vi "ex_GetHeader.vi"(0 "file path":path, 1 "file refs in":T1={"file ref"=refnum, "file size (bytes:0)"=0, "read pointer (bytes:0)"=0, "chunk size (bytes:65000)"=65000}, 2 "file dialog?":bool, 7 "chunk in":string, 9 "first_time?":bool, 11 "error in (no error)":errorcluster) -> (3 "Decimal Separator":string, 4 "hdr special blks":string[](array[string]), 6 "optional info":T3, 8 "file_params":T2 {"time preference" items=["Absolute", "Relative"]; "x_columns" items=["None", "One", "Multiple"]}, 10 "delimiter":string, 12 "chunk remainder":string, 13 "file refs out":T1, 14 "origin timestamp":timestamp format="%<%X\n%x>T", 15 "error out":errorcluster)   [LabVIEW 2020]
uses:
  <vilib>/express/express shared/ExFile.llb/ex_FileReference.ctl
  <vilib>/express/express input/ExFileReadBlock.llb/ex_ReadFileParams.ctl
  <vilib>/express/express shared/ExFile.llb/ex_FileGlobals.vi
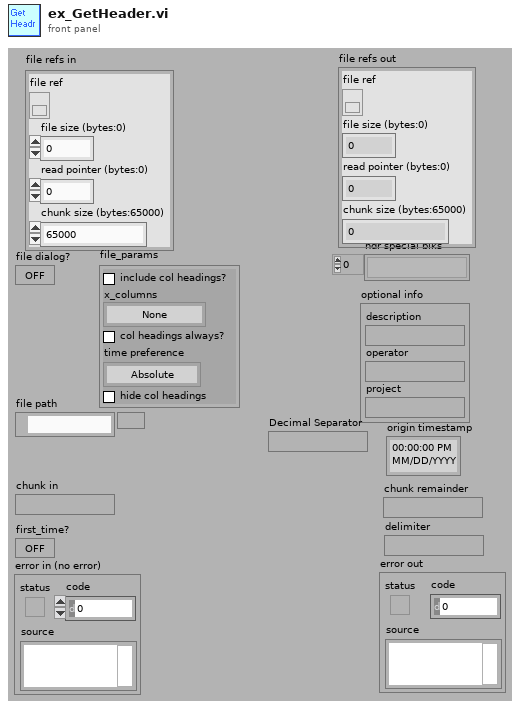
[diagram p1: front panel]
types:
  T1 = typedef "ex_FileReference.ctl" = cluster{"file ref":refnum<file>, "file size (bytes:0)":i32, "read pointer (bytes:0)":i32, "chunk size (bytes:65000)":i32}
  T2 = typedef "ex_ReadFileParams.ctl" = cluster{"include col headings?":bool, "x_columns":u16, "col headings always?":bool, "time preference":u16, "hide col headings":bool}
  T3 = cluster{"description":string, "operator":string, "project":string}
  T4 = enum32{"existing file", "new file", "new or existing file", "existing dir", "new dir", "new or existing dir", "existing file (use LLBs)", "new file (use LLBs)", "new or existing file (use LLBs)", "new or existing file or directory (use LLBs)"}
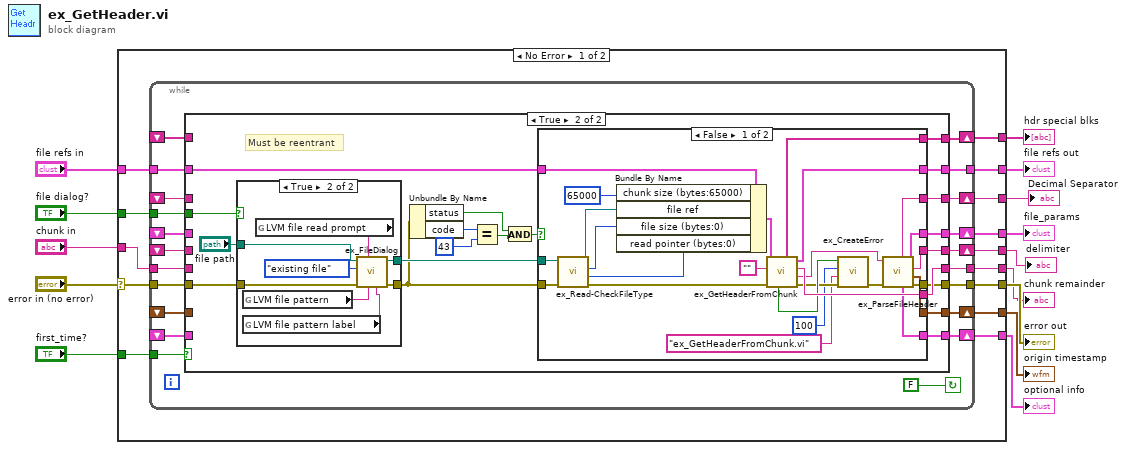
[diagram p0: block diagram]
diagram:
  n1 = case shown="No Error" "error in (no error)" {
    selector: "error in (no error)" -> [w16 w116]
    tunnel: [w28 _] -> w2
    tunnel: [w27 w116] -> w3
    tunnel: [w26 _] -> w4
    tunnel: [w25 _] -> w5
    tunnel: [w24 _] -> w6
    tunnel: [w23 _] -> w7
    tunnel: [w22 _] -> w8
    tunnel: "file refs in" -> [w21 _]
    tunnel: "file dialog?" -> [w20 _]
    tunnel: "first_time?" -> [w19 _]
    tunnel: [w18 _] -> w12
    tunnel: "chunk in" -> [w17 _]
    tunnel: [w15 _] -> w1
    frame No Error {
      n2 = while {
        tunnel: [w49] -> w28
        tunnel: [w48] -> w27
        tunnel: w21 -> [w42]
        tunnel: w16 -> [w41]
        tunnel: w20 -> [w40]
        tunnel: w19 -> [w39]
        shift-right: [w45] -> w24
        shift-left: _ -> [w31]
        shift-right: [w44] -> w23
        shift-left: _ -> [w36]
        shift-right: [w46] -> w25
        shift-left: _ -> [w35]
        shift-right: [w43] -> w22
        shift-left: _ -> [w33]
        shift-right: [w38] -> w18
        shift-left: _ -> [w34]
        tunnel: w17 -> [w32]
        tunnel: [w47] -> w26
        shift-right: [w30] -> w15
        shift-left: _ -> [w29]
        stop <- FALSE continue-if-true
        n3 = case shown="True" w39 {
          tunnel: [w51 w78] -> w49
          tunnel: [w58 w77] -> w48
          tunnel: [w52 w76] -> w47
          tunnel: [w56 w75] -> w46
          tunnel: [w53 w74] -> w45
          tunnel: [w57 w73] -> w44
          tunnel: [w55 w72] -> w38
          tunnel: [w54 w71] -> w43
          tunnel: w42 -> [w52 w66]
          tunnel: w41 -> [w58 w69]
          tunnel: w40 -> [_ w68]
          tunnel: w36 -> [w57 _]
          tunnel: w35 -> [w56 _]
          tunnel: w34 -> [w55 _]
          tunnel: w33 -> [w54 _]
          tunnel: w32 -> [w51 _]
          tunnel: w31 -> [w53 _]
          tunnel: [w50 w65] -> w30
          tunnel: w29 -> [w50 _]
          frame False {
          }
          frame True {
            # "Must be reentrant"
            n4 = case shown="True" w68 {
              tunnel: "file path" -> [w107 w114]
              tunnel: [w107 w113] -> w70
              tunnel: w69 -> [w106 w112]
              tunnel: [w106 w111] -> w64
              frame False {
              }
              frame True {
                n5 = global read "ex_FileGlobals.vi" "LVM file pattern"() -> (w109:string)
                n6 = global read "ex_FileGlobals.vi" "LVM file pattern label"() -> (w108:string)
                n7 = global read "ex_FileGlobals.vi" "LVM file read prompt"() -> (w110:string)
                n8 = call <vilib>:"ex_FileDialog.vi"("pattern label"=w108, "pattern"=w109, "prompt"=w110, "error in (no error)"=w112, "select mode"=T4."existing file", "start path"=w114) -> ("error out"=w111:errorcluster, "selected file path"=w113:path)  [unwired: 4 out]
              }
            }
            n9 = Unbundle By Name(w64) -> ("status"=w60:bool, "code"=w63:i32)
            n10 = Equal?(x=w63, y=43) -> (x = y?=w61:bool)
            n11 = And(x=w60, y=w61) -> (x .and. y?=w59:bool)
            n12 = case shown="False" w59 {
              tunnel: [w103 _] -> w78
              tunnel: [w102 w104] -> w77
              tunnel: [w101 w105] -> w76
              tunnel: [w100 _] -> w75
              tunnel: [w95 _] -> w74
              tunnel: [w94 _] -> w73
              tunnel: [w91 _] -> w72
              tunnel: [w90 _] -> w71
              tunnel: w70 -> [w88 _]
              tunnel: w66 -> [w82 w105]
              tunnel: [w80 _] -> w65
              tunnel: w64 -> [w79 w104]
              frame False {
                n13 = call <vilib>:"ex_Read-CheckFileType.vi"("error in (no error)"=w79, "file path"=w88) -> ("error out"=w96:errorcluster, "mark after read (chars.)"=w93:i32, "file size (bytes)"=w89:i32, "refnum"=w92:refnum<file>)  [unwired: 1 in, 5 out]
                n14 = Bundle By Name(cluster=w82, "chunk size (bytes:65000)"=65000, "file ref"=w92, "file size (bytes:0)"=w89, "read pointer (bytes:0)"=w93) -> (w97:T1)
                n15 = call <vilib>:"ex_GetHeaderFromChunk.vi"("error in (no error)"=w96, "chunk in"="", "file ref in"=w97) -> ("error out"=w86:errorcluster, "header"=w98:string, "chunk remainder"=w103:string, "file ref out"=w101:T1, "special blocks"=w95:string[], "no header?"=w87:bool)  [unwired: 3 out]
                n16 = call <vilib>:"ex_CreateError.vi"("error in (no error)"=w86, "source"="ex_GetHeaderFromChunk.vi", "code"=100, "error?"=w87) -> ("error out"=w85:errorcluster)  [unwired: 7 out]
                n17 = call <vilib>:"ex_ParseFileHeader.vi"("error in (no error)"=w85, "file header string"=w98) -> ("error out"=w102:errorcluster, "Timestamp"=w91:timestamp, "delimiter"=w100:string, "file_params"=w94:T2, "optional info"=w90:T3, "Decimal Separator"=w80:string)  [unwired: 4 out]
              }
              frame True {
              }
            }
          }
        }
      }
    }
    frame Error {
    }
  }
  "origin timestamp" <- w12
  "optional info" <- w8
  "file_params" <- w7
  "hdr special blks" <- w6
  "delimiter" <- w5
  "file refs out" <- w4
  "error out" <- w3
  "chunk remainder" <- w2
  "Decimal Separator" <- w1
